vi "Write Hold.vi"(8 "error in (no error)":errorcluster, 11 "Power Supply in":refnum<class "Power Supply.lvclass">) -> (0 "error out":errorcluster, 3 "Power Supply out":refnum<class "Power Supply.lvclass">)   [LabVIEW 2023, in "Power Supply.lvclass"]
uses:
  Power Supply.lvclass
  Power Supply.lvclass/Power Supply.ctl
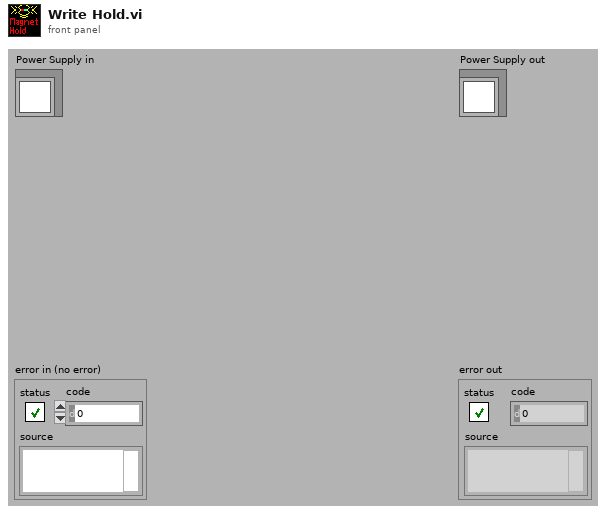
[diagram p1: front panel]
types:
  T1 = typedef "PSIO.ctl" = cluster{"Address":T2, "Version":enum16{"PS", "IPS"}}
  T2 = typedef "OxfordAddress.ctl" = cluster{"Com Port":i32, "ISOBUS Address":i32, "GPIB Address":i16, "Communication":enum16{"RS232", "ISOBUS", "GPIB", "Gateway"}}
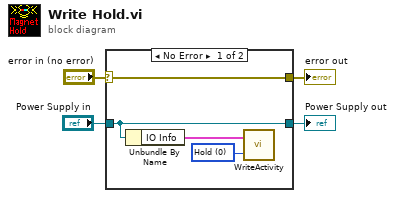
[diagram p0: block diagram]
diagram:
  n1 = case shown="No Error" "error in (no error)" {
    selector: "error in (no error)" -> [w6 w9]
    tunnel: [w5 w10] -> w4
    tunnel: [w6 w9] -> w2
    tunnel: "Power Supply in" -> [w5 w10]
    frame No Error {
      w7 = u16 0 items=["Hold", "To Set Point", "To Zero", "Clamp"] ("Activity")
      n2 = Unbundle By Name(w5) -> ("IO Info"=w8:T1)
      n3 = call "WriteActivity.vi"("Activity"=w7, "IO Info"=w8) -> ()  [unwired: 2 out]
    }
    frame Error {
    }
  }
  "error out" <- w2
  "Power Supply out" <- w4
